vi "createFromDOM.vi"(8 "error in (no error)":errorcluster, 10 "RootElement":refnum<k20>) -> (0 "error out":errorcluster, 3 "NativeXML out":refnum<class "NativeXML.lvclass">)   [LabVIEW 2011, in "Tools.lvlib" / "xml.lvlib" / "NativeXML.lvclass"]
uses:
  NativeXML.lvclass
  NativeXML.lvclass/NativeXML.ctl
  <vilib>/xml/Load XML String.vi
  <vilib>/xml/Close Reference(Node).vi
  <vilib>/xml/NI_XML.lvlib
  Program Files/National Instruments/LabVIEW 2011/resource/objmgr/DOMUserDefRef.rc
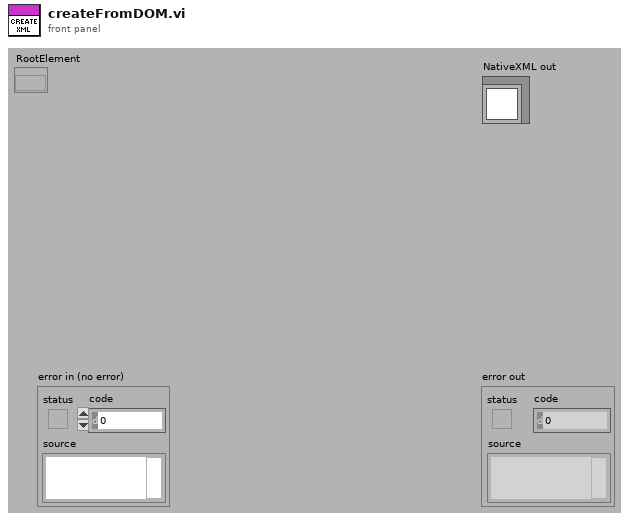
[diagram p1: front panel]
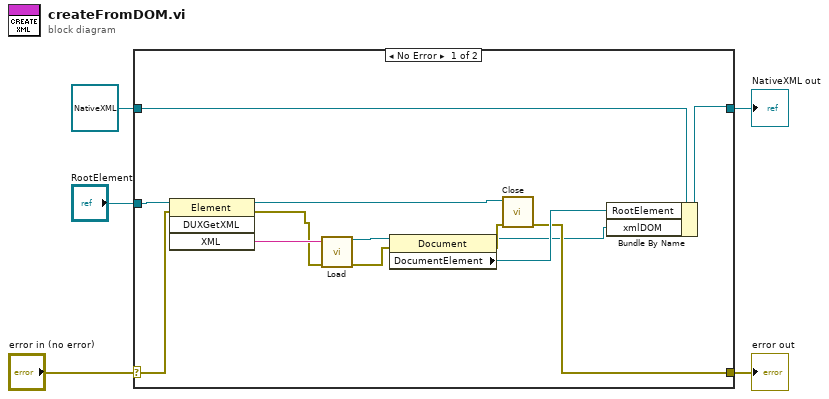
[diagram p0: block diagram]
diagram:
  n1 = case shown="No Error" "error in (no error)" {
    selector: "error in (no error)" -> [w11 w20]
    tunnel: [w7 w20] -> w4
    tunnel: [w17 w19] -> w2
    tunnel: refnum<class "NativeXML.lvclass"> refnum ("NativeXML in") -> [w18 w19]
    tunnel: "RootElement" -> [w14 _]
    frame No Error {
      n2 = invoke class="Element" method="DUXGetXML"(reference=w14, error in=w11) -> (reference out=w9:refnum<k20>, error out=w10:errorcluster, "XML"=w13:string)  [unwired: 2 in, 1 out]
      n3 = call-poly <vilib>:"Load.vi"("XML string"=w13, "error in (no error)"=w10) -> ("DOM document out"=w16:refnum<k20>, "error out"=w15:errorcluster)  [unwired: 11 in, 1 out]
      n4 = property class="Document"(reference=w16, error in=w15) -> (reference out=w6:refnum<k20>, error out=w8:errorcluster, "DocumentElement"=w12:refnum<k20>)
      n5 = call-poly <vilib>:"Close.vi"("error in (no error)"=w8, "node"=w9) -> ("error out"=w7:errorcluster)  [unwired: 7 in]
      n6 = Bundle By Name(cluster=w18, "RootElement"=w12, "xmlDOM"=w6) -> (w17:refnum<class "NativeXML.lvclass">)
    }
    frame Error {
    }
  }
  "error out" <- w4
  "NativeXML out" <- w2
